vi "Initialize2.vi"(8 "error in (no error)":errorcluster, 11 "Sync Box in":refnum<class "Sync Box.lvclass">) -> (0 "error out":errorcluster, 3 "Sync Box out":refnum<class "Sync Box.lvclass">)   [LabVIEW 2012, in "Sync Box.lvclass"]
uses:
  Sync Box.lvclass
  Sync Box.lvclass/Sync Box.ctl
  Comm/Stream/Stream.lvclass
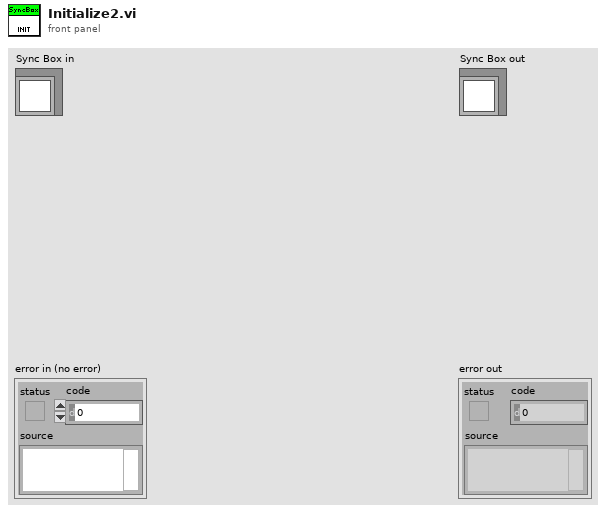
[diagram p1: front panel]
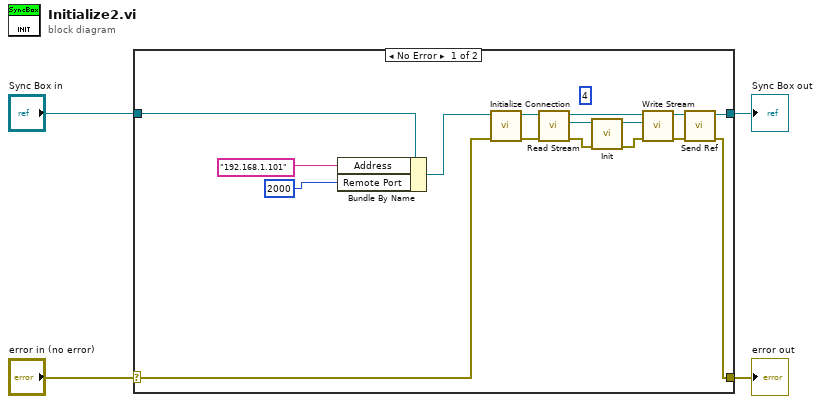
[diagram p0: block diagram]
diagram:
  n1 = case shown="No Error" "error in (no error)" {
    selector: "error in (no error)" -> [w18 w22]
    tunnel: [w11 w22] -> w3
    tunnel: [w7 w21] -> w1
    tunnel: "Sync Box in" -> [w20 w21]
    frame No Error {
      (unwired) u32 4 ("id")
      n2 = Bundle By Name(cluster=w20, "Address"="192.168.1.101" ("Address:"), "Remote Port"=u32 2000 ("Remote Port:")) -> (w19:refnum<class "Sync Box.lvclass">)
      n3 = call "Initialize Connection.vi"("error in (no error)"=w18, "Sync Box in"=w19) -> ("error out"=w9:errorcluster, "Sync Box out"=w10:refnum<class "Sync Box.lvclass">)  [unwired: 8 in]
      n4 = call-dynamic "Read Stream.vi"("error in (no error)"=w9, "Server in"=w10) -> ("error out"=w16:errorcluster, "Stream.lvclass"=w17:refnum<class "Stream.lvclass">, "Server out"=w13:refnum<class "Sync Box.lvclass">)  [unwired: 7 in]
      n5 = call-dynamic "Init.vi"("error in (no error)"=w16, "Stream in"=w17) -> ("error out"=w14:errorcluster, "Stream out"=w15:refnum<class "Stream.lvclass">)  [unwired: 8 in]
      n6 = call-dynamic "Write Stream.vi"("error in (no error)"=w14, "Stream.lvclass"=w15, "Server in"=w13) -> ("error out"=w12:errorcluster, "Server out"=w8:refnum<class "Sync Box.lvclass">)  [unwired: 7 in]
      n7 = call-dynamic "Send Ref.vi"("error in (no error)"=w12, "Sync Box in"=w8) -> ("error out"=w11:errorcluster, "Sync Box out"=w7:refnum<class "Sync Box.lvclass">)  [unwired: 8 in]
    }
    frame Error {
    }
  }
  "error out" <- w3
  "Sync Box out" <- w1
